vi "New__slk_mt.vi"(8 "error in (no error)":errorcluster, 10 "joints":cluster{"X":i32, "Y":i32}[](array[cluster]), 11 "owner refnum in":refnum<vi>) -> (0 "error out":errorcluster, 3 "segment out":refnum<class "Segment__slk_mt.lvclass">)   [LabVIEW 2020, in "Lazyboots Menu Tool.lvlib" / "Segment__slk_mt.lvclass"]
doc: "Creates new segment object by inputing two joints."
uses:
  Segment__slk_mt.lvclass
  TypeDef/TypeDef_Direction__slk_mt.ctl
  Segment__slk_mt.lvclass/Segment__slk_mt.ctl
  Library/Lazyboots Menu Tool.lvlib
panel:
  # "New__slk_mt.vi\nCreates new segment object by inputing two joints.\n\nNOTICE -- YOU MUST LEAVE THIS NOTICE IN PLACE.\n\nCopyright (c) 2011, LIANG LIU Shawn.Liu.cn@gmail.com\nAll rights reserved.\n\nRedistribution and use in source and binary forms, with or without modification, are permitted provided that the following conditions are met:\n-Redistributions of source code must retain the above copyright notice, this list of conditions and the following disclaimer.\n-Redistributions in binary form must reproduce the above copyright notice, this list of conditions and the following disclaimer in the documentation and/or other materials provided with the distribution.\n-Neither the name of the eLp nor the names of its contributors may be used to endorse or promote products derived from this software without specific prior written permission.\n\nTHIS SOFTWARE IS PROVIDED BY THE COPYRIGHT HOLDERS AND CONTRIBUTORS \"AS IS\" AND ANY EXPRESS OR IMPLIED WARRANTIES, INCLUDING, BUT NOT LIMITED TO, THE IMPLIED WARRANTIES OF MERCHANTABILITY AND FITNESS FOR A PARTICULAR PURPOSE ARE DISCLAIMED. IN NO EVENT SHALL THE COPYRIGHT HOLDER OR CONTRIBUTORS BE LIABLE FOR ANY DIRECT, INDIRECT, INCIDENTAL, SPECIAL, EXEMPLARY, OR CONSEQUENTIAL DAMAGES (INCLUDING, BUT NOT LIMITED TO, PROCUREMENT OF SUBSTITUTE GOODS OR SERVICES; LOSS OF USE, DATA, OR PROFITS; OR BUSINESS INTERRUPTION) HOWEVER CAUSED AND ON ANY THEORY OF LIABILITY, WHETHER IN CONTRACT, STRICT LIABILITY, OR TORT (INCLUDING NEGLIGENCE OR OTHERWISE) ARISING IN ANY WAY OUT OF THE USE OF THIS SOFTWARE, EVEN IF ADVISED OF THE POSSIBILITY OF SUCH DAMAGE."
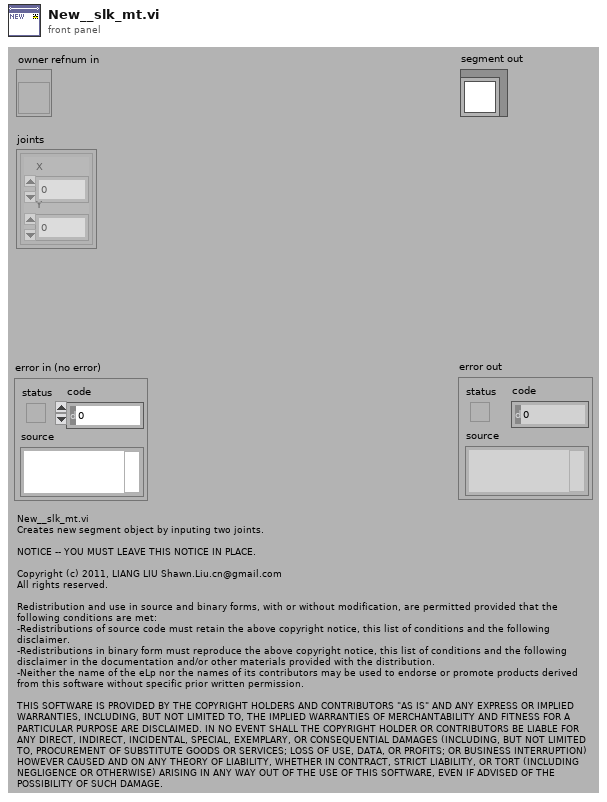
[diagram p1: front panel]
types:
  T1 = typedef "Lazyboots Menu Tool.lvlib/TypeDef_Direction__slk_mt.ctl" = enum16{"Rightward", "Leftward", "Downward", "Upward"}
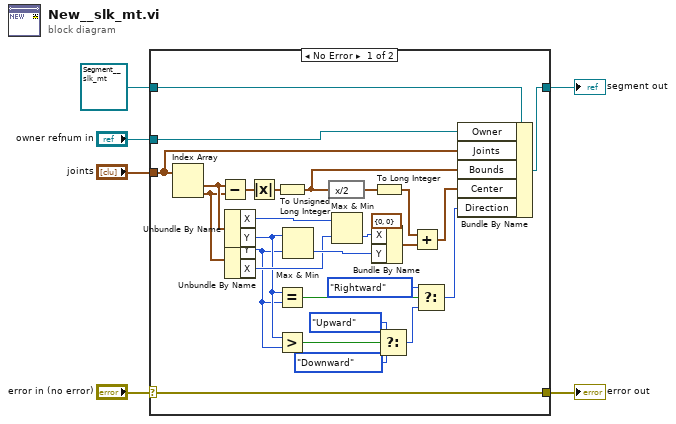
[diagram p0: block diagram]
diagram:
  n1 = case shown="No Error" "error in (no error)" {
    selector: "error in (no error)" -> [w33 w36]
    tunnel: [w33 w36] -> w5
    tunnel: [w32 w35] -> w3
    tunnel: refnum<class "Segment__slk_mt.lvclass"> refnum ("segment in") -> [w34 w35]
    tunnel: "joints" -> [w29 _]
    tunnel: "owner refnum in" -> [w7 _]
    frame No Error {
      n2 = Index Array(array=w29) -> (element #1=w12:cluster{"X":i32, "Y":i32}, element #2=w11:cluster{"X":i32, "Y":i32})  [unwired: 2 in]
      n3 = Subtract(x=w12, y=w11) -> (x-y=w31:cluster{"X":i32, "Y":i32})
      n4 = Unbundle By Name(w12) -> ("X"=w14:i32, "Y"=w10:i32)
      n5 = Unbundle By Name(w11) -> ("Y"=w9:i32, "X"=w15:i32)
      n6 = Absolute Value(x=w31) -> (abs(x)=w30:cluster{"X":i32, "Y":i32})
      n7 = To Unsigned Long Integer(number=w30) -> (unsigned 32bit integer=w13:cluster{"X":u32, "Y":u32})
      n8 = Equal?(x=w10, y=w9) -> (x = y?=w23:bool)
      n9 = Greater?(x=w10, y=w9) -> (0:w25:bool)
      n10 = Max & Min(x=w10, y=w9) -> (min(x,y)=w17:i32)  [unwired: 1 out]
      n11 = expression code="x/2"(w13) -> (w19:cluster{"X":u32, "Y":u32})
      n12 = Max & Min(x=w14, y=w15) -> (min(x,y)=w16:i32)  [unwired: 1 out]
      n13 = Bundle By Name(cluster=cluster{"X":i32, "Y":i32} {"X"=0, "Y"=0} ("Center"), "X"=w16, "Y"=w17) -> (w18:cluster{"X":i32, "Y":i32})
      n14 = To Long Integer(number=w19) -> (32bit integer=w20:cluster{"X":i32, "Y":i32})
      n15 = Select(t=TypeDef_Direction__slk_mt."Upward" ("Direction"), s=w25, f=TypeDef_Direction__slk_mt."Downward" ("Direction")) -> (s? t:f=w24:T1)
      n16 = Add(x=w20, y=w18) -> (x+y=w8:cluster{"X":i32, "Y":i32})
      n17 = Select(t=TypeDef_Direction__slk_mt."Rightward" ("Direction"), s=w23, f=w24) -> (s? t:f=w22:T1)
      n18 = Bundle By Name(cluster=w34, "Owner"=w7, "Joints"=w29, "Bounds"=w13, "Center"=w8, "Direction"=w22) -> (w32:refnum<class "Segment__slk_mt.lvclass">)
    }
    frame Error {
    }
  }
  "error out" <- w5
  "segment out" <- w3
